vi "sub_plot_PDF_in_real_time.vi"(9 "mean":dbl, 10 "variance":dbl, 11 "XYGraph in":refnum<vi>) -> ()   [LabVIEW 2021]
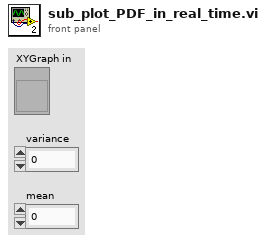
[diagram p1: front panel]
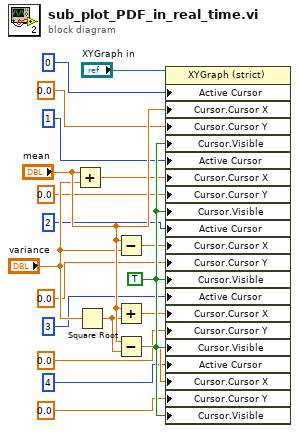
[diagram p0: block diagram]
diagram:
  w16 = TRUE
  n1 = Add(x="mean", y="variance") -> (x+y=w10:dbl)
  n2 = Square Root(x="variance") -> (sqrt(x)=w13:dbl)
  n3 = Subtract(x="mean", y="variance") -> (x-y=w11:dbl)
  n4 = Add(x="mean", y=w13) -> (x+y=w12:dbl)
  n5 = Subtract(x="mean", y=w13) -> (x-y=w14:dbl)
  n6 = property on="Property Node" class="XYGraph (strict)"(reference="XYGraph in", "Active Cursor"=u32 0, "Cursor.Cursor X"="mean", "Cursor.Cursor Y"=0.0 ("Cursor.Cursor Position:Cursor Y"), "Cursor.Visible"=w16, "Active Cursor"=u32 1, "Cursor.Cursor X"=w10, "Cursor.Cursor Y"=0.0 ("Cursor.Cursor Position:Cursor Y"), "Cursor.Visible"=w16, "Active Cursor"=u32 2, "Cursor.Cursor X"=w11, "Cursor.Cursor Y"=0.0 ("Cursor.Cursor Position:Cursor Y"), "Cursor.Visible"=w16, "Active Cursor"=u32 3, "Cursor.Cursor X"=w12, "Cursor.Cursor Y"=0.0 ("Cursor.Cursor Position:Cursor Y"), "Cursor.Visible"=w16, "Active Cursor"=u32 4, "Cursor.Cursor X"=w14, "Cursor.Cursor Y"=0.0 ("Cursor.Cursor Position:Cursor Y"), "Cursor.Visible"=w16) -> ()  [unwired: 1 in, 2 out]
